vi "TRDU_min.vi"() -> ()   [LabVIEW 2020]
panel:
  in  "TRDU_min":dbl
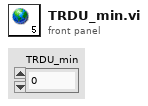
[diagram p1: front panel]
diagram:
